vi "get encoder.vi"(8 "error in (no error)":errorcluster, 10 "zy":i16, 11 "zx":i16) -> (0 "error out":errorcluster, 2 "zy out":i16, 3 "zx out":i16)   [LabVIEW 2015, in "SCANalone4x64.lvlib"]
doc: "__declspec(dllimport) void __stdcall get_encoder(short *zx, short *zy);"
uses:
  <userlib>/SCANalone4x64/SCANalone4x64.lvlib
  <userlib>/SCANalone4x64/SCANalone4x64.dll
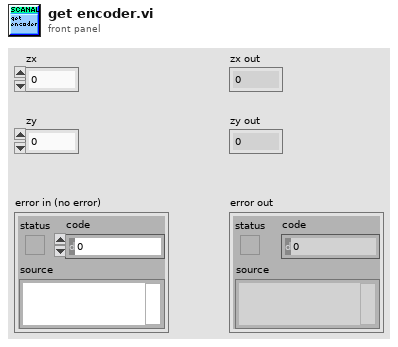
[diagram p1: front panel]
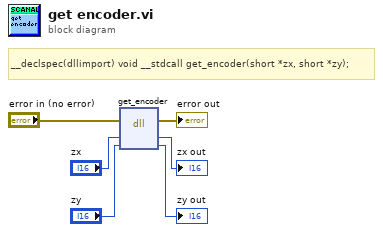
[diagram p0: block diagram]
diagram:
  # "__declspec(dllimport) void __stdcall get_encoder(short *zx, short *zy);"
  n1 = dll-call lib="C:/Program Files/National Instruments/LabVIEW 2015/user.lib/SCANalone4x64/SCANalone4x64.*" fn="get_encoder"(error in="error in (no error)", "zx"="zx", "zy"="zy") -> (error out=→"error out":errorcluster, "zx"=→"zx out":i16, "zy"=→"zy out":i16)  [unwired: 3 in, 1 out]
